vi "integrator.vi"(1 "pretrigger points":u32=1 min=1 step=1, 2 "time":dbl[](array[numeric]) format="%.2f", 3 "input":dbl[](array[numeric]) format="%.3f") -> (0 "output":dbl[](array[numeric]) format="%.9f")   [LabVIEW 2018]
uses:
  <vilib>/Analysis/baseanly.llb/Mean (DBL).vi
  <vilib>/Analysis/NI_AALBase.lvlib
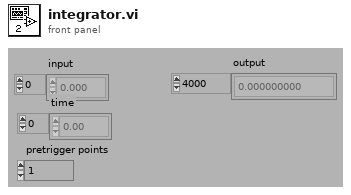
[diagram p1: front panel]
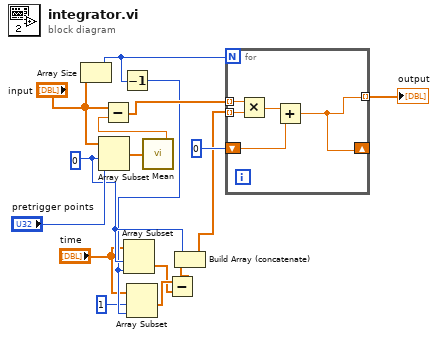
[diagram p0: block diagram]
diagram:
  w8 = 0
  n1 = Array Size(array="input") -> (size(s)=w10:i32)
  n2 = Array Subset(array="input", index=w8, length="pretrigger points") -> (w16:dbl[])
  n3 = Decrement(x=w10) -> (x-1=w7:i32)
  n4 = Array Subset(array="time", index=w8, length=w7) -> (w3:dbl[])
  n5 = Array Subset(array="time", index=1, length=w7) -> (w4:dbl[])
  n6 = call-poly <vilib>:"Mean.vi"("X"=w16) -> ("mean"=w15:dbl)  [unwired: 1 out]
  n7 = Subtract(x="input", y=w15) -> (x-y=w13:dbl[])
  n8 = Subtract(x=w4, y=w3) -> (x-y=w2:dbl[])
  n9 = Build Array (concatenate)(w8, w2) -> (w1:dbl[])
  n10 = for {
    N: w10 -> [_]
    tunnel: w13 -> [w21] mode=indexing
    tunnel: [w17] -> w12 mode=indexing
    shift-right: [w17] -> _
    shift-left: 0 -> [w18]
    tunnel: w1 -> [w20] mode=indexing
    n11 = Multiply(x=w21, y=w20) -> (x*y=w19:dbl)
    n12 = Add(x=w19, y=w18) -> (x+y=w17:dbl)
  }
  "output" <- w12
